vi "Read User configuration.vi"(8 "error in (no error)":errorcluster, 11 "Instrument Driver in":refnum<class "Instrument Driver.lvclass">) -> (0 "error out":errorcluster, 2 "User configuration":variant, 3 "Instrument Driver out":refnum<class "Instrument Driver.lvclass">)   [LabVIEW 2019, in "Instrument Driver.lvclass"]
uses:
  Instrument Driver.lvclass
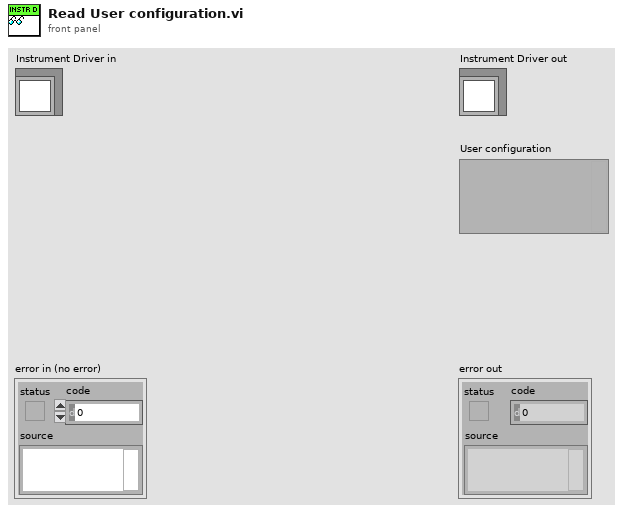
[diagram p1: front panel]
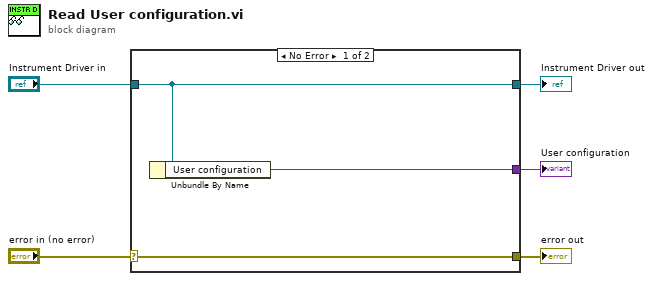
[diagram p0: block diagram]
diagram:
  n1 = case shown="No Error" "error in (no error)" {
    selector: "error in (no error)" -> [w8 w9]
    tunnel: [w8 w9] -> w4
    tunnel: [w7 w10] -> w2
    tunnel: "Instrument Driver in" -> [w7 w10]
    tunnel: [w6 _] -> w1
    frame No Error {
      n2 = Unbundle By Name(w7) -> ("User configuration"=w6:variant)
    }
    frame Error {
    }
  }
  "error out" <- w4
  "Instrument Driver out" <- w2
  "User configuration" <- w1
